vi "Basic Output Character Codes.vi"(8 "error in (no error)":errorcluster, 9 "position (0, 0)":cluster{"row":i8, "column":i8}, 10 "character codes":u8[](array[numeric]), 11 "cluster of class private data in":T1) -> (0 "error out":errorcluster, 1 "current position":cluster{"row":i8, "column":i8}, 3 "cluster of private data out":T1)   [LabVIEW 2017, in "HD44780.lvclass"]
uses:
  HD44780.lvclass
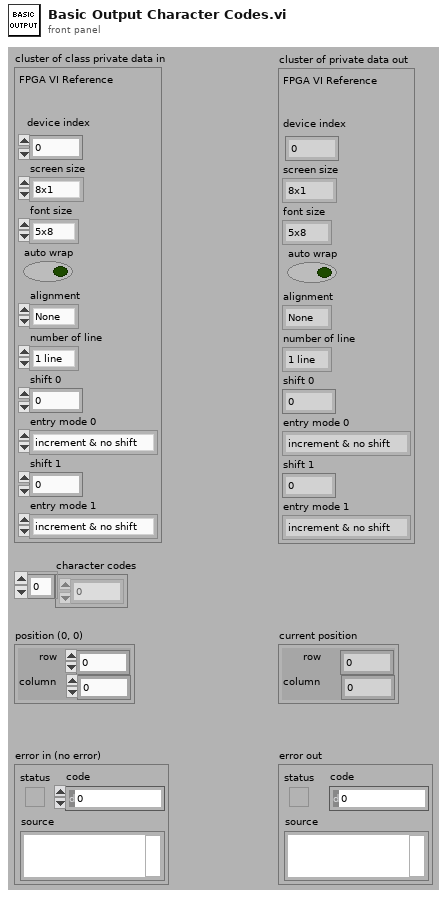
[diagram p1: front panel]
types:
  T1 = cluster{"FPGA VI Reference":refnum<k20>, "device index":i8, "screen size":enum8{"8x1", "8x2", "12x4", "16x1", "16x2", "16x4", "20x1", "20x2", "20x4", "24x1", "24x2", "40x2", "40x4"}, "font size":enum8{"5x8", "5x10"}, "auto wrap":bool, "alignment":enum16{"None", "Left", "Center", "Right"}, "number of line":enum8{"1 line", "2 lines"}, "shift 0":i8, "entry mode 0":enum8{"increment & no shift", "increment & shift", "decrement & no shift", "decrement & shift"}, "shift 1":i8, "entry mode 1":enum8{"increment & no shift", "increment & shift", "decrement & no shift", "decrement & shift"}}
  T2 = enum8{"increment & no shift", "increment & shift", "decrement & no shift", "decrement & shift"}
  T3 = enum8{"increment & no shift", "increment & shift", "decrement & no shift", "decrement & shift"}[]
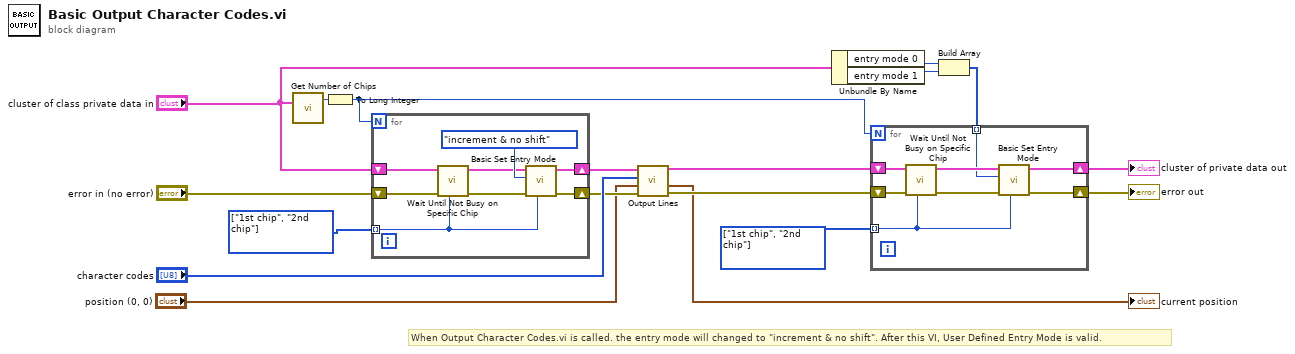
[diagram p0: block diagram]
diagram:
  w12 = enum16{"1st chip", "2nd chip"}[] [enum."1st chip", enum."2nd chip"] items=["1st chip", "2nd chip"] ("initialized array")
  w10 = enum16{"1st chip", "2nd chip"}[] [enum."1st chip", enum."2nd chip"] items=["1st chip", "2nd chip"] ("initialized array")
  # "When Output Character Codes.vi is called. the entry mode will changed to \"increment & no shift\". After this VI, User Defined Entry Mode is valid."
  n1 = call "Get Number of Chips.vi"("cluster of private data in"="cluster of class private data in") -> ("number of chips"=w9:u8)  [unwired: 10 in]
  n2 = To Long Integer(number=w9) -> (32bit integer=w5:i32)
  n3 = for {
    N: w5 -> [_]
    tunnel: w10 -> [w19] mode=indexing
    shift-right: [w24] -> w2
    shift-left: "error in (no error)" -> [w23]
    shift-right: [w25] -> w3
    shift-left: "cluster of class private data in" -> [w22]
    n4 = call "Wait Until Not Busy on Specific Chip.vi"("chip select  (1st chip)"=w19, "error in (no error)"=w23, "cluster of private data in"=w22) -> ("error out"=w21:errorcluster, "cluster of private data out"=w20:T1)  [unwired: 7 in]
    n5 = call "Basic Set Entry Mode.vi"("chip select  (1st chip)"=w19, "error in (no error)"=w21, "entry mode (increment & no shift)"=T2."increment & no shift" ("entry mode"), "cluster of private data in"=w20) -> ("error out"=w24:errorcluster, "cluster of private data out"=w25:T1)  [unwired: 6 in]
  }
  n6 = call "Output Lines.vi"("error in (no error)"=w2, "position (0, 0)"="position (0, 0)", "character codes"="character codes", "cluster of private data in"=w3) -> ("error out"=w6:errorcluster, "current position"=→"current position":cluster{"row":i8, "column":i8}, "cluster of private data out"=w7:T1)  [unwired: 4 in]
  n7 = Unbundle By Name("cluster of class private data in") -> ("entry mode 0"=w13:T2, "entry mode 1"=w14:T2)
  n8 = Build Array(w13, w14) -> (w15:T3)
  n9 = for {
    N: w5 -> [_]
    tunnel: w12 -> [w27] mode=indexing
    shift-right: [w28] -> w16
    shift-left: w6 -> [w33]
    tunnel: w15 -> [w30] mode=indexing
    shift-right: [w29] -> w11
    shift-left: w7 -> [w34]
    n10 = call "Wait Until Not Busy on Specific Chip.vi"("chip select  (1st chip)"=w27, "error in (no error)"=w33, "cluster of private data in"=w34) -> ("error out"=w32:errorcluster, "cluster of private data out"=w31:T1)  [unwired: 7 in]
    n11 = call "Basic Set Entry Mode.vi"("chip select  (1st chip)"=w27, "error in (no error)"=w32, "entry mode (increment & no shift)"=w30, "cluster of private data in"=w31) -> ("error out"=w28:errorcluster, "cluster of private data out"=w29:T1)  [unwired: 6 in]
  }
  "error out" <- w16
  "cluster of private data out" <- w11
